vi "Shoot_Sequence.vi"(10 "Start?":bool) -> ()   [LabVIEW 2019]
uses:
  <vilib>/Rock Robotics/WPI/ThirdParty/Phoenix-LabVIEW/Motor Controller/Controls/CTRE_Phoenix_MotorControl_ControlMode.ctl
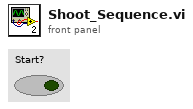
[diagram p1: front panel]
types:
  T1 = typedef "WPI_MotorControlDeviceRef.ctl" = cluster{"DeviceStatus":errorcluster, "Type":T2, "PWM":cluster{"PWM Channel":T3, "DeadBand":T4}, "CAN":cluster{"Device Number":u8, "SetOutput VI Ref":variant, "GetOutput VI Ref":variant, "Enable VI Ref":variant, "Disable VI Ref":variant, "Data":variant}, "Invert":bool, "DIO PWM":cluster{"PWM \"Enable\" Channel":T3, "DIOChannel":T5, "PWM Rate":dbl}}
  T2 = typedef "WPI_MotorControlType.ctl" = enum16{"PWM", "CAN", "DIO PWM"}
  T3 = typedef "FPGA_DIOPWMChannel.ctl" = enum8{"PWM 0", "PWM 1", "PWM 2", "PWM 3", "PWM 4", "PWM 5", "PWM 6", "PWM 7", "PWM 8", "PWM 9", "PWM MXP 0", "PWM MXP 1", "PWM MXP 2", "PWM MXP 3", "PWM MXP 4", "PWM MXP 5", "PWM MXP 6", "PWM MXP 7", "PWM MXP 8", "PWM MXP 9", "Invalid"}
  T4 = typedef "WPI_PWMDeadband.ctl" = cluster{"Name":string, "maxPositivePwm":i32, "minPositivePwm":i32, "centerPwm":i32, "maxNegativePwm":i32, "minNegativePwm":i32, "angularRange":u16}
  T5 = typedef "FPGA_DIOChannel.ctl" = enum8{"DIO 0", "DIO 1", "DIO 2", "DIO 3", "DIO 4", "DIO 5", "DIO 6", "DIO 7", "DIO 8", "DIO 9", "DIO MXP 0", "DIO MXP 1", "DIO MXP 2", "DIO MXP 3", "DIO MXP 4", "DIO MXP 5", "DIO MXP 6", "DIO MXP 7", "DIO MXP 8", "DIO MXP 9", "DIO MXP 10", "DIO MXP 11", "DIO MXP 12", "DIO MXP 13", "DIO MXP 14", "DIO MXP 15", "SPI Port CS1", "SPI Port CS2", "SPI Port CS3", "SPI Port MISO", "SPI Port MOSI", "Invalid"}
  T6 = typedef "CTRE_Phoenix_MotorControl_ControlMode.ctl" = u16
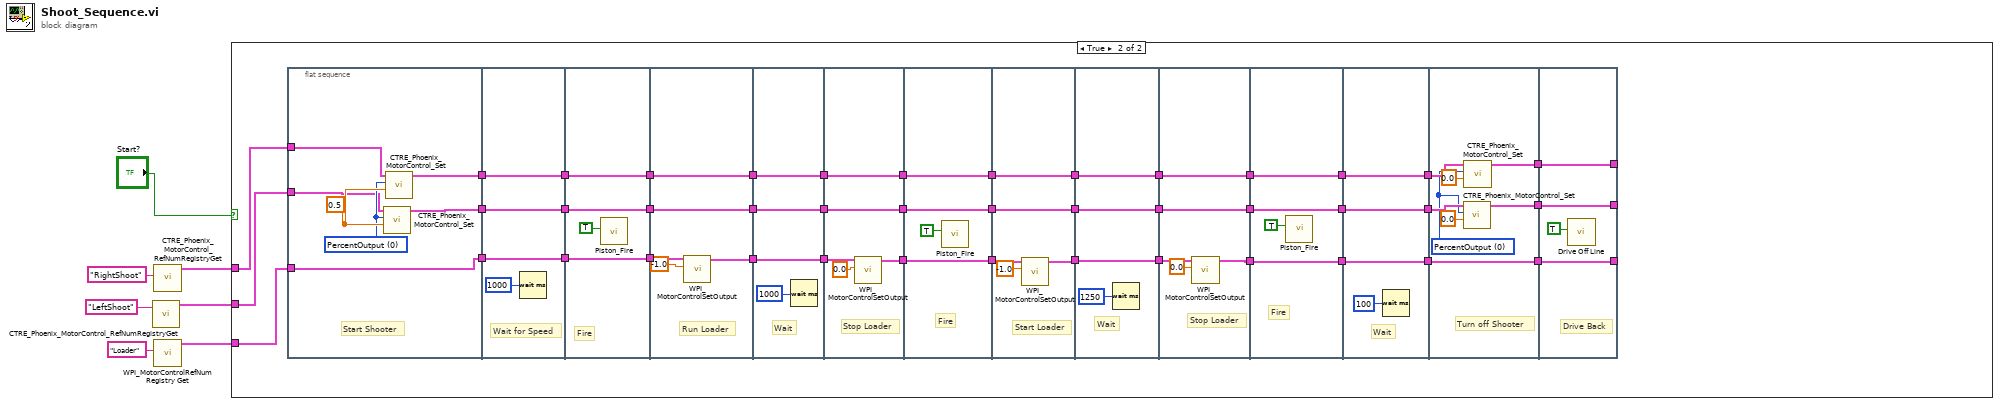
[diagram p0: block diagram]
diagram:
  n1 = call <vilib>:"CTRE_Phoenix_MotorControl_RefNumRegistryGet.vi"("refnum name"="LeftShoot") -> ("PhoenixMotorControlDevRef"=w2:T1)  [unwired: 9 in, 1 out]
  n2 = call <vilib>:"CTRE_Phoenix_MotorControl_RefNumRegistryGet.vi"("refnum name"="RightShoot") -> ("PhoenixMotorControlDevRef"=w1:T1)  [unwired: 9 in, 1 out]
  n3 = call <vilib>:"WPI_MotorControlRefNum Registry Get.vi"("refnum name"="Loader") -> ("MotorControlDevRef"=w3:T1)  [unwired: 9 in, 1 out]
  n4 = case shown="True" "Start?" {
    tunnel: w3 -> [_ w10]
    tunnel: w2 -> [_ w9]
    tunnel: w1 -> [_ w8]
    frame False {
    }
    frame True {
      n5 = flat-sequence {
        tunnel: [w52] -> w49
        tunnel: [w55] -> w48
        tunnel: [w54] -> w47
        tunnel: w10 -> [w52]
        tunnel: w9 -> [w51]
        tunnel: w8 -> [w50]
        tunnel: w49 -> [w60]
        tunnel: w48 -> [w59]
        tunnel: w47 -> [w58]
        tunnel: [w60] -> w46
        tunnel: [w59] -> w45
        tunnel: [w58] -> w44
        tunnel: w46 -> [w64]
        tunnel: w45 -> [w63]
        tunnel: w44 -> [w62]
        tunnel: [w64] -> w43
        tunnel: [w63] -> w42
        tunnel: [w62] -> w41
        tunnel: w43 -> [w67]
        tunnel: w42 -> [w69]
        tunnel: w41 -> [w68]
        tunnel: [w69] -> w40
        tunnel: [w68] -> w39
        tunnel: [w65] -> w38
        tunnel: w40 -> [w73]
        tunnel: w39 -> [w72]
        tunnel: w38 -> [w70]
        tunnel: [w73] -> w37
        tunnel: [w72] -> w36
        tunnel: [w70] -> w35
        tunnel: w37 -> [w78]
        tunnel: w36 -> [w77]
        tunnel: w35 -> [w76]
        tunnel: [w78] -> w34
        tunnel: [w77] -> w33
        tunnel: [w75] -> w32
        tunnel: w34 -> [w82]
        tunnel: w33 -> [w81]
        tunnel: w32 -> [w80]
        tunnel: [w82] -> w31
        tunnel: [w81] -> w30
        tunnel: [w80] -> w29
        tunnel: w31 -> [w87]
        tunnel: w30 -> [w86]
        tunnel: w29 -> [w84]
        tunnel: [w87] -> w28
        tunnel: [w86] -> w27
        tunnel: [w85] -> w26
        tunnel: w28 -> [w91]
        tunnel: w27 -> [w90]
        tunnel: w26 -> [w89]
        tunnel: [w91] -> w25
        tunnel: [w90] -> w24
        tunnel: [w89] -> w23
        tunnel: w25 -> [w96]
        tunnel: w24 -> [w95]
        tunnel: w23 -> [w94]
        tunnel: [w96] -> w22
        tunnel: [w95] -> w21
        tunnel: [w93] -> w20
        tunnel: w22 -> [w100]
        tunnel: w21 -> [w99]
        tunnel: w20 -> [w98]
        tunnel: [w100] -> w19
        tunnel: [w99] -> w18
        tunnel: [w98] -> w17
        tunnel: w19 -> [w104]
        tunnel: w18 -> [w103]
        tunnel: w17 -> [w102]
        tunnel: [w104] -> w16
        tunnel: [w103] -> w15
        tunnel: [w102] -> w14
        tunnel: w16 -> [w111]
        tunnel: w15 -> [w110]
        tunnel: w14 -> [w112]
        tunnel: [w112] -> w13
        tunnel: [w107] -> w12
        tunnel: [w106] -> w11
        tunnel: [w114] -> _
        tunnel: [w115] -> _
        tunnel: [w116] -> _
        tunnel: w13 -> [w116]
        tunnel: w12 -> [w115]
        tunnel: w11 -> [w114]
        frame #0 {
          w53 = T6 0 items=["PercentOutput"=0, "Position"=1, "Velocity"=2, "Current"=3, "Follower"=5, "MotionProfile"=6, "MotionMagic"=7, "MotionProfileArc"=10, "Disabled"=15] ("Control Mode")
          w56 = 0.5 ("Output")
          # "Start Shooter"
          n6 = call <vilib>:"CTRE_Phoenix_MotorControl_Set.vi"("Output"=w56, "Control Mode"=w53, "PhoenixMotorControlDevRef"=w51) -> ("PhoenixMotorControlDevRef"=w54:T1)  [unwired: 7 in, 1 out]
          n7 = call <vilib>:"CTRE_Phoenix_MotorControl_Set.vi"("Output"=w56, "Control Mode"=w53, "PhoenixMotorControlDevRef"=w50) -> ("PhoenixMotorControlDevRef"=w55:T1)  [unwired: 7 in, 1 out]
        }
        frame #1 {
          # "Wait for Speed"
          n8 = Wait (ms)(milliseconds to wait=u32 1000) -> ()  [unwired: 1 out]
        }
        frame #2 {
          # "Fire"
          n9 = call "Piston_Fire.vi"("Fire?"=TRUE) -> ()  [unwired: 11 in]
        }
        frame #3 {
          # "Run Loader"
          n10 = call <vilib>:"WPI_MotorControlSetOutput.vi"("Output"=-1.0, "MotorControlDevRef"=w67) -> ("MotorControlDevRef"=w65:T1)  [unwired: 7 in, 2 out]
        }
        frame #4 {
          # "Wait"
          n11 = Wait (ms)(milliseconds to wait=u32 1000) -> ()  [unwired: 1 out]
        }
        frame #5 {
          # "Stop Loader"
          n12 = call <vilib>:"WPI_MotorControlSetOutput.vi"("Output"=0.0, "MotorControlDevRef"=w76) -> ("MotorControlDevRef"=w75:T1)  [unwired: 7 in, 2 out]
        }
        frame #6 {
          # "Fire"
          n13 = call "Piston_Fire.vi"("Fire?"=TRUE) -> ()  [unwired: 11 in]
        }
        frame #7 {
          # "Start Loader"
          n14 = call <vilib>:"WPI_MotorControlSetOutput.vi"("Output"=-1.0, "MotorControlDevRef"=w84) -> ("MotorControlDevRef"=w85:T1)  [unwired: 7 in, 2 out]
        }
        frame #8 {
          # "Wait"
          n15 = Wait (ms)(milliseconds to wait=u32 1250) -> ()  [unwired: 1 out]
        }
        frame #9 {
          # "Stop Loader"
          n16 = call <vilib>:"WPI_MotorControlSetOutput.vi"("Output"=0.0, "MotorControlDevRef"=w94) -> ("MotorControlDevRef"=w93:T1)  [unwired: 7 in, 2 out]
        }
        frame #10 {
          # "Fire"
          n17 = call "Piston_Fire.vi"("Fire?"=TRUE) -> ()  [unwired: 11 in]
        }
        frame #11 {
          # "Wait"
          n18 = Wait (ms)(milliseconds to wait=u32 100) -> ()  [unwired: 1 out]
        }
        frame #12 {
          w105 = T6 0 items=["PercentOutput"=0, "Position"=1, "Velocity"=2, "Current"=3, "Follower"=5, "MotionProfile"=6, "MotionMagic"=7, "MotionProfileArc"=10, "Disabled"=15] ("Control Mode")
          # "Turn off Shooter"
          n19 = call <vilib>:"CTRE_Phoenix_MotorControl_Set.vi"("Output"=0.0, "Control Mode"=w105, "PhoenixMotorControlDevRef"=w110) -> ("PhoenixMotorControlDevRef"=w107:T1)  [unwired: 7 in, 1 out]
          n20 = call <vilib>:"CTRE_Phoenix_MotorControl_Set.vi"("Output"=0.0, "Control Mode"=w105, "PhoenixMotorControlDevRef"=w111) -> ("PhoenixMotorControlDevRef"=w106:T1)  [unwired: 7 in, 1 out]
        }
        frame #13 {
          # "Drive Back"
          n21 = call "Drive Off Line.vi"("Start?"=TRUE) -> ()  [unwired: 11 in]
        }
      }
    }
  }
